vi "sender-receiver-udp.vi"() -> ()   [LabVIEW 2017]
panel:
  in  "TargetAngles":dbl[](array[numeric])
  in  "String?":bool
  in  "Enum":T1(ring)
  in  "data in":string="qqq"
  out "Array":dbl[](array[numeric])
  in  "Stop":bool
  out "Received Data":dbl(graph)
  out "data out":string
  out "rest of the binary string":string
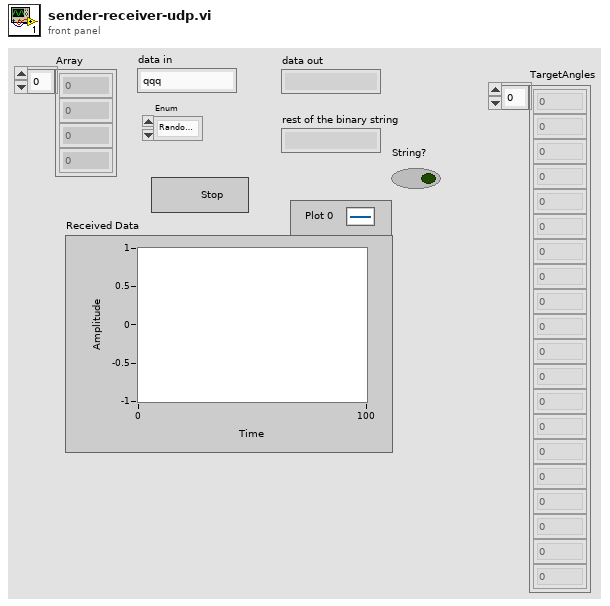
[diagram p1: front panel]
types:
  T1 = enum16{"RandomNumber", "Text", "Random Array", "Sinusoid"}
  T2 = enum16{"big-endian, network order", "native, host order", "little-endian"}
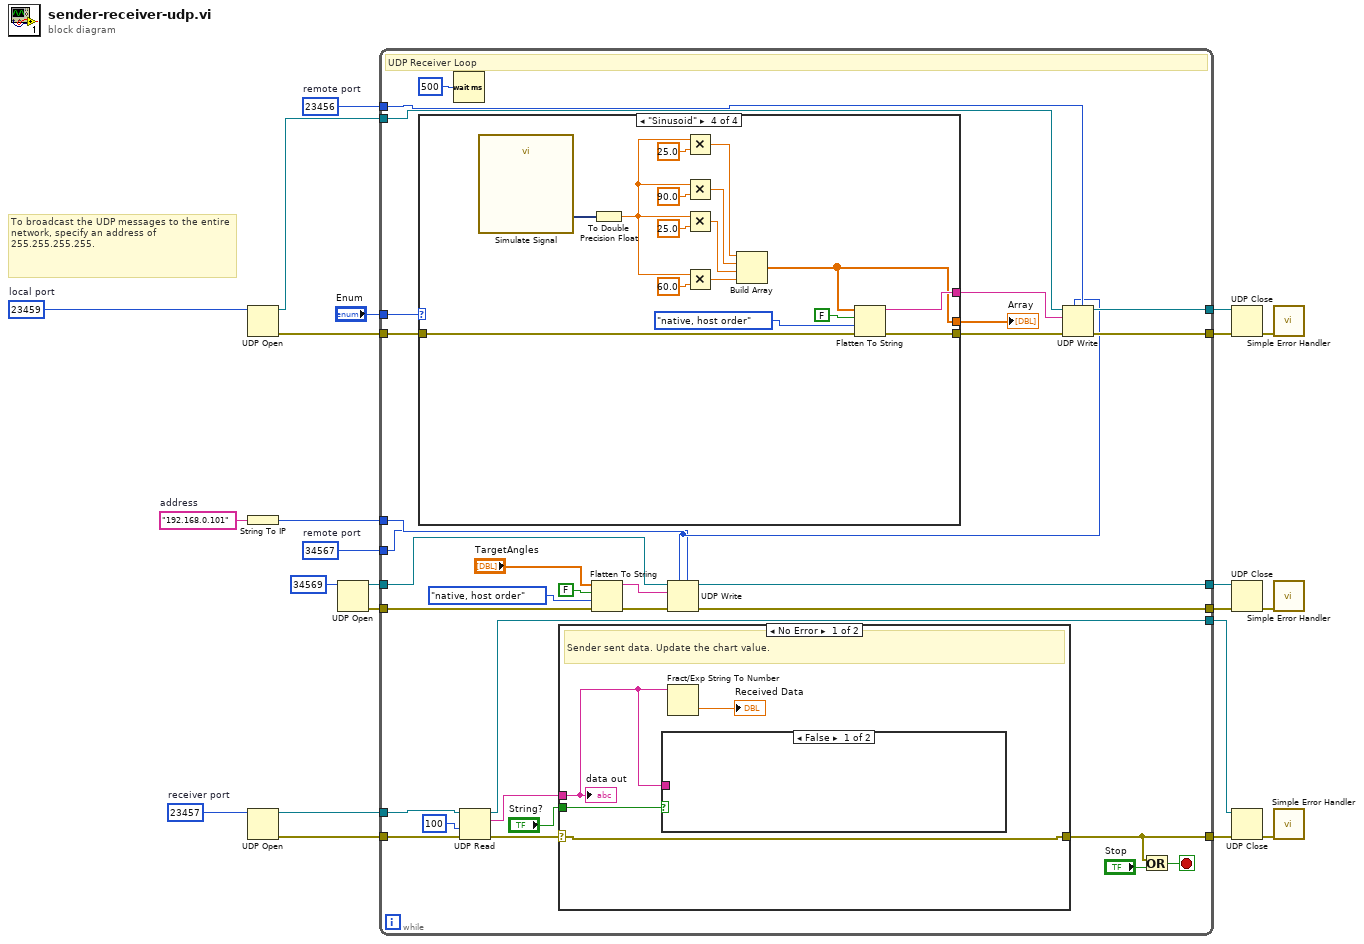
[diagram p0: block diagram]
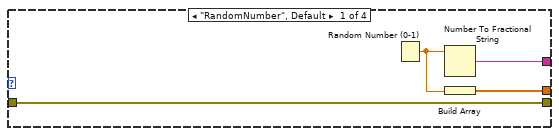
[diagram p2: hidden frame]
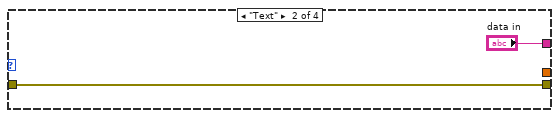
[diagram p3: hidden frame]
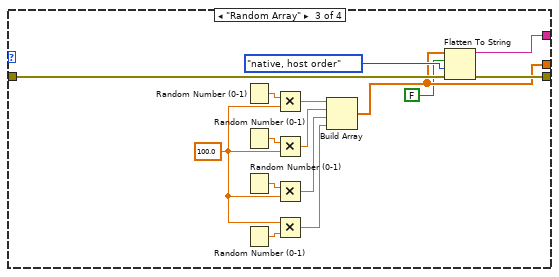
[diagram p4: hidden frame]
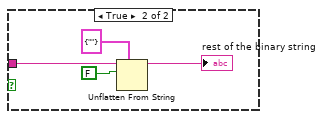
[diagram p5: hidden frame]
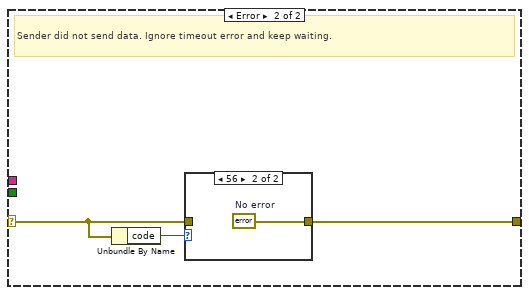
[diagram p6: hidden frame]
diagram:
  w4 = u16 34567  # remote port
  w15 = u16 23456  # remote port
  w16 = u16 23459  # local port
  w18 = "192.168.0.101"  # address
  w19 = u16 23457  # receiver port
  # "To broadcast the UDP messages to the entire network, specify an address of 255.255.255.255."
  n1 = UDP Open(11:w16) -> (port=w13:refnum<k16>, 0:w9:errorcluster)  [unwired: 4 in, 1 out]
  n2 = String To IP(1:w18) -> (0:w14:u32)
  n3 = UDP Open(11:w19) -> (port=w20:refnum<k16>, 0:w21:errorcluster)  [unwired: 4 in, 1 out]
  n4 = UDP Open(11:u16 34569 ("port")) -> (port=w5:refnum<k16>, 0:w6:errorcluster)  [unwired: 4 in, 1 out]
  n5 = while {
    tunnel: w20 -> [w54]
    tunnel: [w47] -> w23
    tunnel: w21 -> [w52]
    tunnel: [w48] -> w8
    tunnel: w15 -> [w43]
    tunnel: w14 -> [w28]
    tunnel: w13 -> [w42]
    tunnel: [w41] -> w12
    tunnel: [w40] -> w11
    tunnel: "Enum" -> [w39]
    tunnel: w9 -> [w38]
    tunnel: w6 -> [w31]
    tunnel: w5 -> [w30]
    tunnel: w4 -> [w27]
    tunnel: [w25] -> w2
    tunnel: [w24] -> w1
    stop <- w53 stop-if-true
    # "UDP Receiver Loop"
    n6 = case shown="\"Sinusoid\"" w39 {
      tunnel: [w57 "data in" w70 w84] -> w37
      tunnel: w38 -> [w58 w59 w69 w81]
      tunnel: [w58 w59 w68 w83] -> w36
      tunnel: [w55 _ w67 w82] -> w35
      frame "RandomNumber", Default {
        n7 = Random Number (0-1)() -> (number: 0 to 1=w56:dbl)
        n8 = Number To Fractional String(number=w56) -> (F-format string=w57:string)  [unwired: 3 in]
        n9 = Build Array(w56) -> (w55:dbl[])
      }
      frame "Text" {
      }
      frame "Random Array" {
        w62 = 100.0 ("y")
        n10 = Random Number (0-1)() -> (number: 0 to 1=w75:dbl)
        n11 = Random Number (0-1)() -> (number: 0 to 1=w74:dbl)
        n12 = Random Number (0-1)() -> (number: 0 to 1=w73:dbl)
        n13 = Random Number (0-1)() -> (number: 0 to 1=w72:dbl)
        n14 = Multiply(x=w75, y=w62) -> (x*y=w66:dbl)
        n15 = Multiply(x=w74, y=w62) -> (x*y=w65:dbl)
        n16 = Multiply(x=w73, y=w62) -> (x*y=w64:dbl)
        n17 = Multiply(x=w62, y=w72) -> (x*y=w63:dbl)
        n18 = Build Array(w66, w65, w64, w63) -> (w67:dbl[])
        n19 = Flatten To String(anything=w67, prepend array or string size? (T)=FALSE, byte order (0:big-endian, network order)=T2."native, host order", error in (no error)=w69) -> (data string=w70:string, error out=w68:errorcluster)  [unwired: 1 out]
      }
      frame "Sinusoid" {
        n20 = call "Simulate Signal"() -> ("Sine"=w80:dynamicdata)  [unwired: 14 in, 1 out]
        n21 = To Double Precision Float(number=w80) -> (double precision float=w78:dbl)
        n22 = Multiply(x=w78, y=25.0) -> (x*y=w90:dbl)
        n23 = Multiply(x=w78, y=90.0) -> (x*y=w89:dbl)
        n24 = Multiply(x=w78, y=25.0) -> (x*y=w88:dbl)
        n25 = Multiply(x=w78, y=60.0) -> (x*y=w87:dbl)
        n26 = Build Array(w90, w89, w88, w87) -> (w82:dbl[])
        n27 = Flatten To String(anything=w82, prepend array or string size? (T)=FALSE, byte order (0:big-endian, network order)=T2."native, host order", error in (no error)=w81) -> (data string=w84:string, error out=w83:errorcluster)  [unwired: 1 out]
      }
    }
    "Array" <- w35
    n28 = Wait (ms)(milliseconds to wait=u32 500) -> ()  [unwired: 1 out]
    n29 = UDP Read(connection ID=w54, timeout ms (25000)=100, 8:w52) -> (data out=w50:string, error out=w49:errorcluster, 3:w47:refnum<k16>)  [unwired: 3 out]
    n30 = case shown="No Error" w49 {
      selector: w49 -> [w94 w101]
      tunnel: w50 -> [w93 _]
      tunnel: [w94 w100] -> w48
      tunnel: "String?" -> [w92 _]
      frame No Error {
        # "Sender sent data. Update the chart value."
        n31 = case shown="False" w92 {
          tunnel: w93 -> [_ w98]
          frame False {
          }
          frame True {
            n32 = Unflatten From String(type=cluster{string} {""}, binary string=w98, data includes array or string size? (T)=FALSE) -> (rest of the binary string=→"rest of the binary string":string)  [unwired: 2 in, 2 out]
          }
        }
        n33 = Fract/Exp String To Number(string=w93) -> (number=→"Received Data":dbl)  [unwired: 3 in, 1 out]
        "data out" <- w93
      }
      frame Error {
        # "Sender did not send data. Ignore timeout error and keep waiting."
        n34 = Unbundle By Name(w101) -> ("code"=w102:i32)
        n35 = case shown="56" w102 {
          tunnel: w101 -> [w103 _]
          tunnel: [w103 w104] -> w100
          frame Default {
          }
          frame 56 {
            w104 = errorcluster {"status"=FALSE, "code"=0, "source"=""}  # No error
          }
        }
      }
    }
    n36 = Flatten To String(anything="TargetAngles", prepend array or string size? (T)=FALSE, byte order (0:big-endian, network order)=T2."native, host order", error in (no error)=w31) -> (data string=w29:string, error out=w26:errorcluster)  [unwired: 1 out]
    n37 = UDP Write(address=w28, port or service name=w27, connection ID=w30, data in=w29, 8:w26) -> (error out=w25:errorcluster, 3:w24:refnum<k16>)  [unwired: 1 in]
    n38 = UDP Write(address=w28, port or service name=w43, connection ID=w42, data in=w37, 8:w36) -> (error out=w41:errorcluster, 3:w40:refnum<k16>)  [unwired: 1 in]
    n39 = Or(x=w48, y="Stop") -> (x .or. y?=w53:bool)
  }
  n40 = UDP Close(connection ID=w11, 8:w12) -> (error out=w17:errorcluster)  [unwired: 1 out]
  n41 = UDP Close(connection ID=w1, 8:w2) -> (error out=w3:errorcluster)  [unwired: 1 out]
  n42 = UDP Close(connection ID=w23, 8:w8) -> (error out=w22:errorcluster)  [unwired: 1 out]
  n43 = call <vilib>:"Simple Error Handler.vi"("error in (no error)"=w17) -> ()  [unwired: 4 in, 5 out]
  n44 = call <vilib>:"Simple Error Handler.vi"("error in (no error)"=w3) -> ()  [unwired: 1 in, 8 out]
  n45 = call <vilib>:"Simple Error Handler.vi"("error in (no error)"=w22) -> ()  [unwired: 1 in, 8 out]
